vi "Decorate.vi"(10 "Event":refnum<class "Event.lvclass">, 11 "eeeee in":refnum<class "eeeee.lvclass">) -> (3 "eeeee out":refnum<class "eeeee.lvclass">)   [LabVIEW 2021, in "jettl Tools.lvlib" / "eeeee.lvlib" / "eeeee.lvclass"]
uses:
  eeeee.lvclass
  jettl/Event/Event.lvclass
  eeeee.lvclass/eeeee.ctl
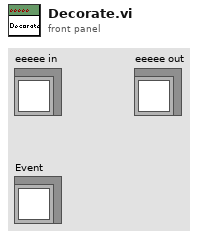
[diagram p1: front panel]
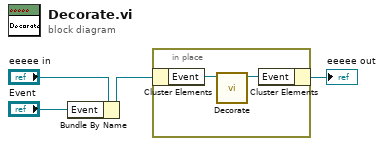
[diagram p0: block diagram]
diagram:
  n1 = Bundle By Name(cluster="eeeee in", "Event"="Event") -> (w2:refnum<class "eeeee.lvclass">)
  n2 = in-place {
    n3 = in-place-cluster #1(w2) -> ("Event"=w6:refnum<class "Event.lvclass">)
    n4 = call-dynamic "Decorate.vi"("Event in"=w6) -> ("Event out"=w5:refnum<class "Event.lvclass">)  [unwired: 10 in]
    n5 = in-place-cluster #1("Event"=w5) -> (→"eeeee out":refnum<class "eeeee.lvclass">)
  }
